vi "MotorGetNamed.vi"(0 "Motor status in":T1={"Managed?"=FALSE, "Position"=0, "Name"="unknown", "Status"=enum."OFF"}, 1 "MotorName":string, 2 "MotorData":T2[](array[typedef])) -> (3 "Motor status out":T1={"Managed?"=FALSE, "Position"=0, "Name"="unknown", "Status"=enum."OFF"})   [LabVIEW 2009]
uses:
  Controls/MotorData.ctl
  Controls/MotorNamedPosition.ctl
  Controls/MotorStatus.ctl
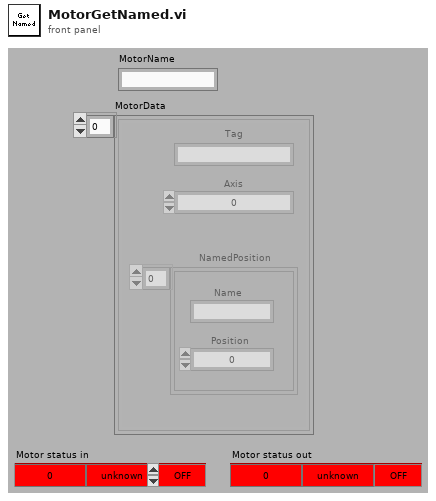
[diagram p1: front panel]
types:
  T1 = typedef "MotorStatus.ctl" = cluster{"Managed?":bool, "Position":i32, "Name":string, "Status":enum16{"OFF", "IDLE", "MOVING", "HOMING"}}
  T2 = typedef "MotorData.ctl" = cluster{"Tag":string, "Axis":i32, "NamedPosition":T3[]}
  T3 = typedef "MotorNamedPosition.ctl" = cluster{"Position":i32, "Name":string}
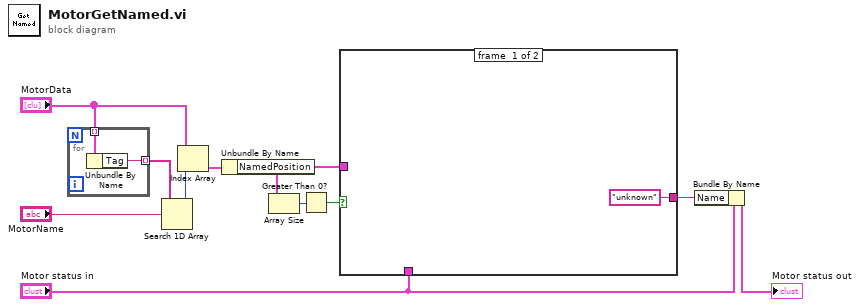
[diagram p0: block diagram]
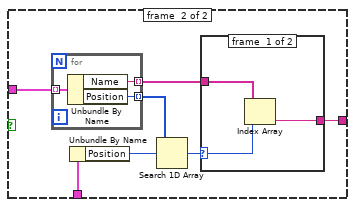
[diagram p2: hidden frame]
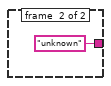
[diagram p3: hidden frame]
diagram:
  n1 = for {
    tunnel: [w13] -> w11 mode=indexing
    tunnel: "MotorData" -> [w12] mode=indexing
    n2 = Unbundle By Name(w12) -> ("Tag"=w13:string)
  }
  n3 = Search 1D Array(1D array=w11, element="MotorName") -> (index of element=w9:i32)  [unwired: 1 out]
  n4 = Index Array(array="MotorData", index=w9) -> (element=w7:T2)
  n5 = Unbundle By Name(w7) -> ("NamedPosition"=w3:T3[])
  n6 = Array Size(array=w3) -> (size(s)=w2:i32)
  n7 = Greater Than 0?(x=w2) -> (x > 0?=w1:bool)
  n8 = case shown="True" w1 {
    tunnel: w3 -> [_ w21]
    tunnel: ["unknown" ("Name") w17] -> w6
    tunnel: "Motor status in" -> [_ w16]
    frame #0 {
    }
    frame #1 {
      n9 = for {
        tunnel: w21 -> [w28] mode=indexing
        tunnel: [w27] -> w18 mode=indexing
        tunnel: [w26] -> w20 mode=indexing
        n10 = Unbundle By Name(w28) -> ("Name"=w27:string, "Position"=w26:i32)
      }
      n11 = Unbundle By Name(w16) -> ("Position"=w19:i32)
      n12 = Search 1D Array(1D array=w20, element=w19) -> (index of element=w15:i32)  [unwired: 1 out]
      n13 = case shown="0, Default" w15 {
        selector: w15 -> [w22 _]
        tunnel: w18 -> [w24 _]
        tunnel: [w23 "unknown" ("Name")] -> w17
        frame #0 {
          n14 = Index Array(array=w24, index=w22) -> (element=w23:string)
        }
        frame #1 {
        }
      }
    }
  }
  n15 = Bundle By Name(cluster="Motor status in", "Name"=w6) -> (→"Motor status out":T1)
